vi "air_pump_ch.vi"() -> ()   [LabVIEW 2019]
uses:
  FSM_NEO-PP2.ctl
panel:
  in  "Tab Control":enum32{"Settings", "Measurements", "Analysis"}(tab)
  out "Voltage Limit [V]":dbl
  out "Current Limit [A]":dbl
  in  "address GPIB":string(combo)
  in  "DC Voltage [V]":dbl(slide) min=0.0 max=12.0 step=12.0 scale=0.0..12.0
  in  "DC Current MAX [A]":dbl(slide)=0.6 min=0.6 max=1.0 step=0.005 scale=0.6..1.0
  in  "ENABLE":bool
  in  "DISPLAY":bool
  in  "CLEAR AND RESET":bool
  in  "Output Channel":enum32{"Item 0", "Item 1", "Radio Selection 3"}(radio)
  in  "OUTPUT":bool
  in  "DC CURRENT [mA]":dbl(knob) min=0.0 max=1000.0 step=50.0 scale=0.0..1000.0
  out "?":string
  out "Waveform Graph":dbl[](graph)
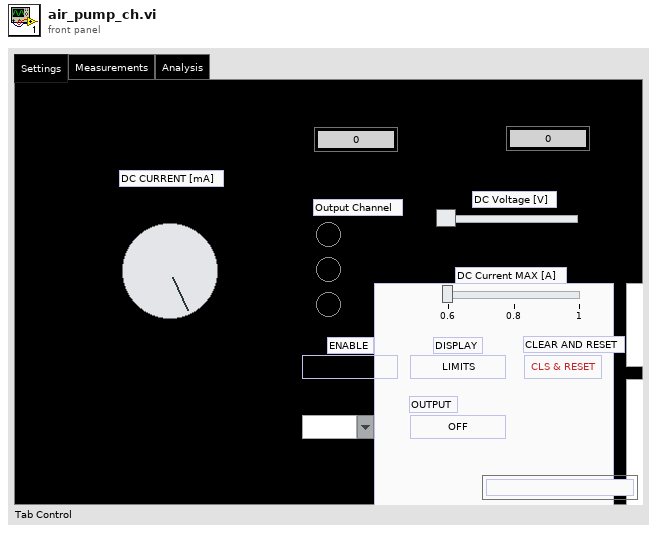
[diagram p1: front panel]
types:
  T1 = typedef "FSM_NEO-PP2.ctl" = enum16{"limit_mode", "meter_mode", "error", "display_limits", "beep", "clear_error", "change_output", "select_ch", "remote", "output", "idle", "start"}
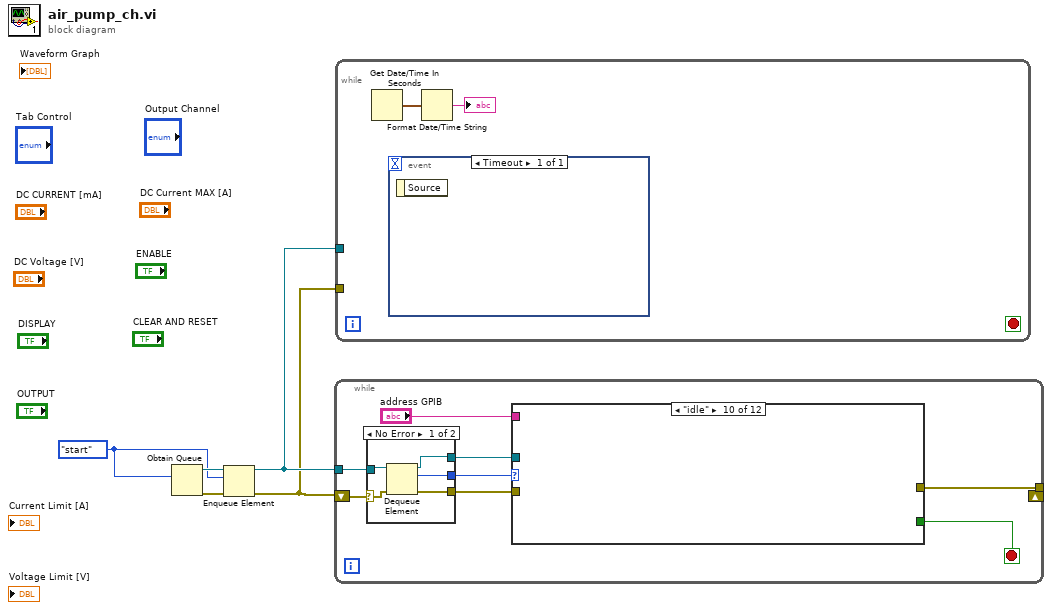
[diagram p0: block diagram]
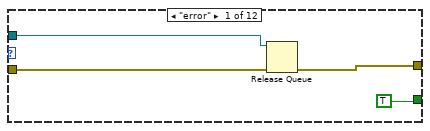
[diagram p2: hidden frame]
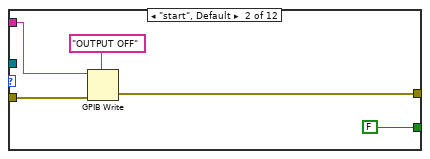
[diagram p3: hidden frame]
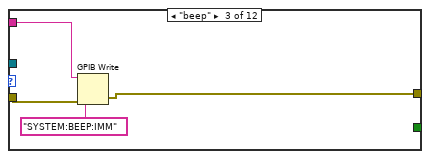
[diagram p4: hidden frame]
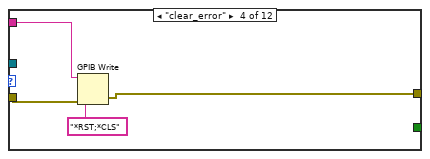
[diagram p5: hidden frame]
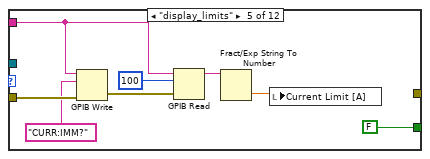
[diagram p6: hidden frame]
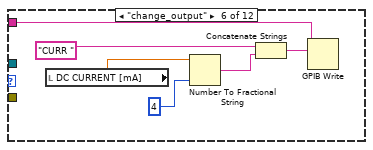
[diagram p7: hidden frame]
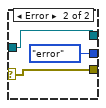
[diagram p13: hidden frame]
diagram:
  w3 = FSM_NEO-PP2."start" ("Enum")
  n1 = Obtain Queue(element data type=w3) -> (queue out=w5:refnum<queue>, error out=w4:errorcluster)  [unwired: 4 in, 1 out]
  n2 = Enqueue Element(queue=w5, element=w3, error in (no error)=w4) -> (queue out=w2:refnum<queue>, error out=w1:errorcluster)  [unwired: 1 in, 1 out]
  n3 = while {
    tunnel: w2 -> [w12]
    tunnel: [w9] -> _
    shift-right: _ -> [_]
    shift-left: w1 -> [w13]
    stop <- w6 stop-if-true
    n4 = case shown="No Error" w13 {
      selector: w13 -> [w49 w51]
      tunnel: w12 -> [w48 w50]
      tunnel: [w47 w51] -> w11
      tunnel: [w46 FSM_NEO-PP2."error" ("Enum")] -> w8
      tunnel: [w45 w50] -> w10
      frame No Error {
        n5 = Dequeue Element(queue=w48, error in (no error)=w49) -> (queue out=w45:refnum<queue>, element=w46:T1, error out=w47:errorcluster)  [unwired: 1 in, 1 out]
      }
      frame Error {
      }
    }
    n6 = case shown="\"idle\"" w8 {
      tunnel: w11 -> [w17 w21 w25 w29 w38 _ _ _ _ _ _ _]
      tunnel: w10 -> [w16 _ _ _ _ _ _ _ _ _ _ _]
      tunnel: [w15 w19 w23 w27 _ _ _ _ _ _ _ _] -> w9
      tunnel: "address GPIB" -> [_ w22 w26 w30 w35 w44 _ _ _ _ _ _]
      tunnel: [TRUE FALSE _ _ FALSE _ _ _ _ _ _ _] -> w6
      frame "error" {
        n7 = Release Queue(queue=w16, error in (no error)=w17) -> (error out=w15:errorcluster)  [unwired: 1 in, 2 out]
      }
      frame "start", Default {
        n8 = GPIB Write(0:w22, 1:"OUTPUT OFF" ("data"), 3:w21) -> (6:w19:errorcluster)  [unwired: 2 in, 1 out]
      }
      frame "beep" {
        n9 = GPIB Write(0:w26, 1:"SYSTEM:BEEP:IMM" ("data"), 3:w25) -> (6:w23:errorcluster)  [unwired: 2 in, 1 out]
      }
      frame "clear_error" {
        n10 = GPIB Write(0:w30, 1:"*RST;*CLS" ("data"), 3:w29) -> (6:w27:errorcluster)  [unwired: 2 in, 1 out]
      }
      frame "display_limits" {
        n11 = GPIB Write(0:w35, 1:"CURR:IMM?" ("data"), 3:w38) -> (6:w34:errorcluster)  [unwired: 2 in, 1 out]
        n12 = GPIB Read(0:w35, 1:100 ("byte count"), 3:w34) -> (5:w32:string)  [unwired: 2 in, 2 out]
        n13 = Fract/Exp String To Number(string=w32) -> (number=w31:dbl)  [unwired: 3 in, 1 out]
        n14 = local write "Current Limit [A]"(w31) -> ()
      }
      frame "change_output" {
        n15 = local read "DC CURRENT [mA]"() -> (w43:dbl)
        n16 = Number To Fractional String(number=w43, precision (6)=i16 4) -> (F-format string=w40:string)  [unwired: 2 in]
        n17 = Concatenate Strings("CURR " ("data"), w40) -> (w42:string)
        n18 = GPIB Write(0:w44, 1:w42) -> ()  [unwired: 3 in, 2 out]
      }
      frame "select_ch" {
      }
      frame "remote" {
      }
      frame "output" {
      }
      frame "idle" {
      }
      frame "meter_mode" {
      }
      frame "limit_mode" {
      }
    }
  }
  n19 = while {
    tunnel: w2 -> [_]
    tunnel: w1 -> [_]
    stop <- _ stop-if-true
    n20 = Get Date/Time In Seconds() -> (seconds since 1Jan1904=w54:timestamp)
    n21 = event shown="[0] Timeout" {
      selector: _ -> [_]
      dyn-events: _ -> [_]
      timeout: _ -> [_]
      event Timeout {
        n22 = event-data() -> ()  [unwired: 1 in, 1 out]
      }
    }
    n23 = Format Date/Time String(seconds (now)=w54) -> (date/time string=→"?":string)  [unwired: 2 in]
  }
